vi "gbtp.vi"(5 "x":dbl, 6 "p":dbl[](array[numeric])) -> (2 "f(x;p)":dbl)   [LabVIEW 2021]
doc: "Sum of three Gaussians, plus DC offset."
panel:
  # "I0\nmu\nw\nI1"
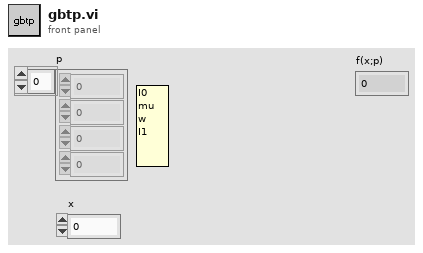
[diagram p1: front panel]
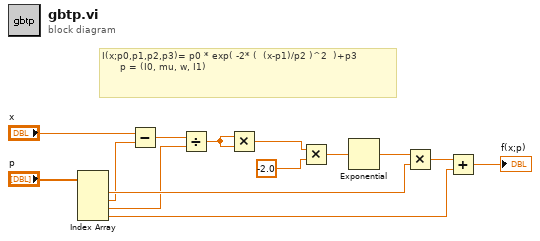
[diagram p0: block diagram]
diagram:
  # "I(x;p0,p1,p2,p3)= p0 * exp( -2* (  (x-p1)/p2 )^2  )+p3\n      p = (I0, mu, w, I1)"
  n1 = Index Array(array="p") -> (element #1=w4:dbl, element #2=w3:dbl, element #3=w2:dbl, element #4=w1:dbl)  [unwired: 4 in]
  n2 = Subtract(x="x", y=w3) -> (x-y=w12:dbl)
  n3 = Divide(x=w12, y=w2) -> (x/y=w11:dbl)
  n4 = Multiply(x=w11, y=w11) -> (x*y=w10:dbl)
  n5 = Multiply(x=w10, y=-2.0) -> (x*y=w9:dbl)
  n6 = Exponential(1:w9) -> (0:w5:dbl)
  n7 = Multiply(x=w5, y=w4) -> (x*y=w6:dbl)
  n8 = Add(x=w6, y=w1) -> (x+y=→"f(x;p)":dbl)
